vi "XBrio write test2 (int to fracitonal string).vi"() -> ()   [LabVIEW 2013]
uses:
  C:/Program Files (x86)/National Instruments/LabVIEW 2013/examples/Instrument IO/Serial/support/Serial - Settings.ctl
  <vilib>/Instr/_visa.llb/VISA Configure Serial Port (Instr).vi
panel:
  out "String being written in HEX":string
  out "String being written":string
  in  "Number being sent":u8
  out "Bytes being written":u32
  in  "Numeric input 2":i32
  in  "Numeric input":i32
  in  "VISA resource name":refnum<visa-resource-name>="COM1"
  in  "delay before read (ms)":u32=500
  out "bytes read":u32
  in  "Serial Settings":T1={"baud rate"=9600, "data bits"=8, "parity"=enum."None", "stop bits"=10, "flow control"=0} {"flow control" items=["None"=0, "XON/XOFF"=1, "RTS/CTS"=2, "DTR/DSR"=4]; "stop bits" items=["1.0"=10, "1.5"=15, "2.0"=20]; "data bits" min=5 max=8 step=1; "baud rate" items=["75"=75, "110"=110, "134"=134, "150"=150, "300"=300, "600"=600, "1200"=1200, "1800"=1800, "2400"=2400, "4800"=4800, "7200"=7200, "9600"=9600, "14400"=14400, "19200"=19200, "28800"=28800, "38400"=38400, "56000"=56000, "57600"=57600, "115200"=115200, "128000"=128000, "230400"=230400]}
  in  "?":bool
  out "Response":string
  out "String to U16":u16[](array[numeric])
  out "IR2":u16
  out "IR1":u16
  out "Encoder1":u16
  out "Encoder2":u16
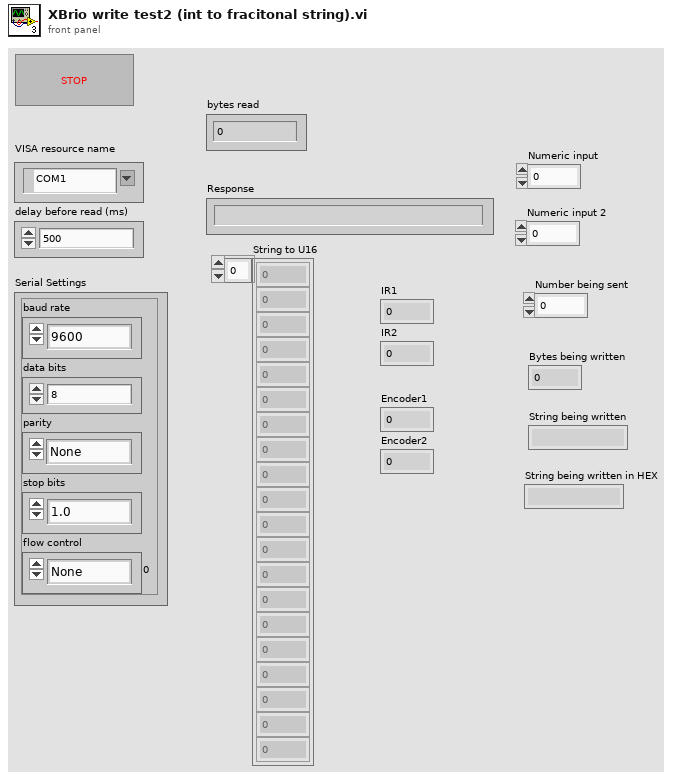
[diagram p1: front panel]
types:
  T1 = typedef "Serial - Settings.ctl" = cluster{"baud rate":u32, "data bits":u16, "parity":enum16{"None", "Odd", "Even", "Mark", "Space"}, "stop bits":u16, "flow control":u16}
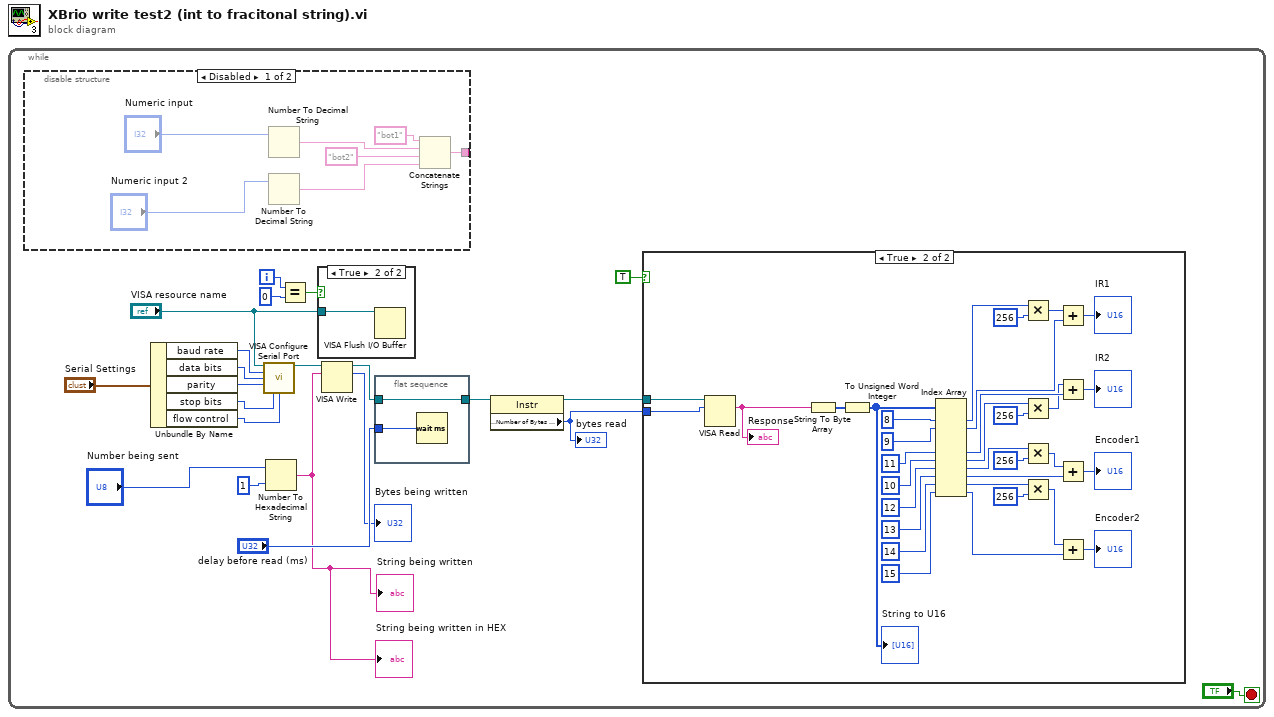
[diagram p0: block diagram]
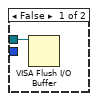
[diagram p3: hidden frame]
diagram:
  n1 = while {
    i -> [w13]
    stop <- "?" stop-if-true
    n2 = disable-structure shown="Disabled" {
      disable-tunnel: [w23 _] -> _
      frame Disabled {
        n3 = Number To Decimal String(number="Numeric input") -> (decimal integer string=w26:string)  [unwired: 1 in]
        n4 = Number To Decimal String(number="Numeric input 2") -> (decimal integer string=w27:string)  [unwired: 1 in]
        n5 = Concatenate Strings("bot1" ("string"), w26, "bot2" ("string"), w27) -> (w23:string)
      }
      frame Enabled {
      }
    }
    n6 = Unbundle By Name("Serial Settings") -> ("baud rate"=w20:u32, "data bits"=w19:u16, "parity"=w18:enum16{"None", "Odd", "Even", "Mark", "Space"}, "stop bits"=w17:u16, "flow control"=w16:u16)
    n7 = call-poly "VISA Configure Serial Port"("VISA resource name"="VISA resource name", "baud rate (9600)"=w20, "data bits (8)"=w19, "parity (0:none)"=w18, "stop bits (10: 1 bit)"=w17, "flow control (0:none)"=w16) -> ("VISA resource name out"=w7:refnum<visa-resource-name>)  [unwired: 3 in, 6 out]
    n8 = Number To Hexadecimal String(1:u8 1 ("width (-)"), 2:"Number being sent") -> (0:w2:string)
    "String being written" <- w2
    "String being written in HEX" <- w2
    n9 = Equal?(x=w13, y=0) -> (x = y?=w11:bool)
    n10 = case shown="True" w11 {
      tunnel: "VISA resource name" -> [_ w64]
      frame False {
      }
      frame True {
        n11 = VISA Flush I/O Buffer(VISA resource name=w64) -> ()  [unwired: 2 in, 2 out]
      }
    }
    n12 = VISA Write(VISA resource name=w7, write buffer=w2) -> (VISA resource name out=w6:refnum<visa-resource-name>, return count=→"Bytes being written":u32)  [unwired: 1 in, 1 out]
    n13 = flat-sequence {
      tunnel: w6 -> [w65]
      tunnel: [w65] -> w15
      tunnel: "delay before read (ms)" -> [w66]
      frame #0 {
        n14 = Wait (ms)(milliseconds to wait=w66) -> ()  [unwired: 1 out]
      }
    }
    n15 = property class="Instr"(reference=w15) -> (reference out=w8:refnum<visa-resource-name>, "Serial Settings:Number of Bytes at Serial Port"=w9:u32)  [unwired: 1 in, 1 out]
    "bytes read" <- w9
    n16 = case shown="True" TRUE {
      tunnel: w9 -> [_ w32]
      tunnel: w8 -> [w30 w31]
      frame False {
        n17 = VISA Flush I/O Buffer(VISA resource name=w30) -> ()  [unwired: 2 in, 2 out]
      }
      frame True {
        n18 = VISA Read(VISA resource name=w31, byte count=w32) -> (read buffer=w34:string)  [unwired: 1 in, 3 out]
        "Response" <- w34
        n19 = String To Byte Array(string=w34) -> (unsigned byte array=w35:u8[])
        n20 = To Unsigned Word Integer(number=w35) -> (unsigned 16bit integer=w33:u16[])
        "String to U16" <- w33
        n21 = Index Array(array=w33, index #1=8 ("index"), index #2=9 ("index"), index #5=11, index #6=10 ("index"), index #7=12 ("index"), index #8=13 ("index"), index #9=14 ("index"), index #10=15 ("index")) -> (element #1=w43:u16, element #2=w46:u16, element #5=w40:u16, element #6=w38:u16, element #7=w51:u16, element #8=w52:u16, element #9=w58:u16, element #10=w59:u16)  [unwired: 2 in, 2 out]
        n22 = Multiply(x=w43, y=u16 256) -> (x*y=w45:u16)
        n23 = Multiply(x=w38, y=u16 256) -> (x*y=w36:u16)
        n24 = Multiply(x=w51, y=u16 256) -> (x*y=w47:u16)
        n25 = Multiply(x=w58, y=u16 256) -> (x*y=w57:u16)
        n26 = Add(x=w45, y=w46) -> (x+y=→"IR1":u16)
        n27 = Add(x=w36, y=w40) -> (x+y=→"IR2":u16)
        n28 = Add(x=w47, y=w52) -> (x+y=→"Encoder1":u16)
        n29 = Add(x=w57, y=w59) -> (x+y=→"Encoder2":u16)
      }
    }
  }
